vi "saveLogEntry.vi"(8 "error in (no error)":errorcluster, 11 "Logger in":refnum<class "TestDataLog.lvclass">) -> (0 "error out":errorcluster, 3 "Logger out":refnum<class "TestDataLog.lvclass">)   [LabVIEW 2015, in "TestDataLog.lvclass"]
uses:
  TestDataLog.lvclass
  TestDataLog.lvclass/TestDataLog.ctl
  <userlib>/Common/Log/Log/Log.lvclass/Log.ctl
  <userlib>/Common/Log/Log/Log.lvclass
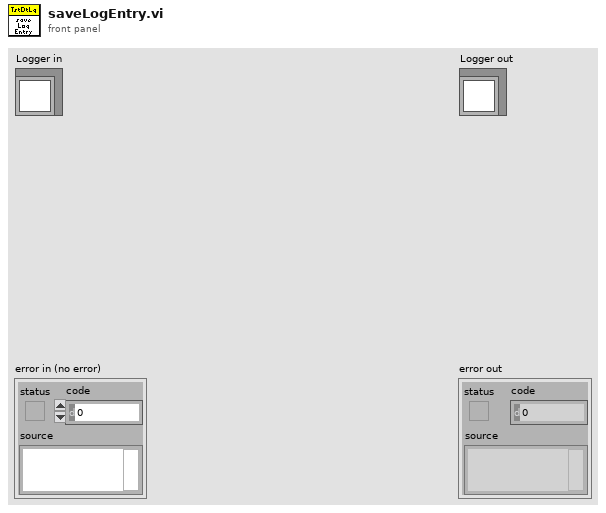
[diagram p1: front panel]
types:
  T1 = typedef "M1M3SSSTypedefs.lvlib/InputData.ctl" = cluster{"Force Measured":T2, "Distance Data":T3}
  T2 = typedef "M1M3SSSTypedefs.lvlib/ForceDemand.ctl" = dbl[unit]
  T3 = typedef "DistanceGauge.lvlib/Distance Data.ctl" = cluster{"Distance Measured 1":dbl[unit], "Distance Measured 2":dbl[unit]}
  T4 = typedef "M1M3SSSTypedefs.lvlib/OutputData.ctl" = cluster{"Ramp Output":u16}
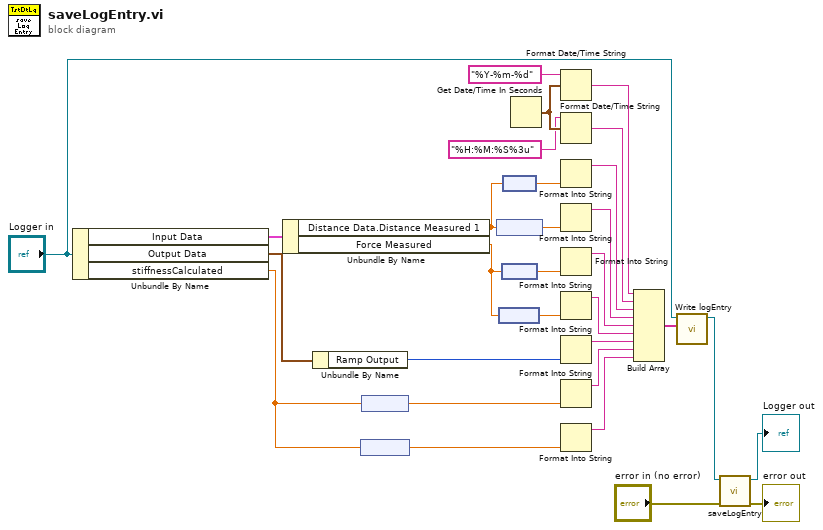
[diagram p0: block diagram]
diagram:
  n1 = Unbundle By Name("Logger in") -> ("Input Data"=w30:T1, "Output Data"=w29:T4, "stiffnessCalculated"=w2:dbl[unit])
  n2 = Unbundle By Name(w30) -> ("Distance Data.Distance Measured 1"=w8:dbl[unit], "Force Measured"=w5:T2)
  n3 = Unbundle By Name(w29) -> ("Ramp Output"=w28:u16)
  n4 = node(w2) -> (w12:dbl)
  n5 = node(w2) -> (w3:dbl)
  n6 = node(w8) -> (w25:dbl)
  n7 = node(w5) -> (w6:dbl)
  n8 = node(w5) -> (w26:dbl)
  n9 = node(w8) -> (w10:dbl)
  n10 = Get Date/Time In Seconds() -> (seconds since 1Jan1904=w24:timestamp)
  n11 = Format Date/Time String(time format string (%c)="%Y-%m-%d" ("format string"), seconds (now)=w24) -> (date/time string=w21:string)  [unwired: 1 in]
  n12 = Format Date/Time String(time format string (%c)="%H:%M:%S%3u", seconds (now)=w24) -> (date/time string=w22:string)  [unwired: 1 in]
  n13 = Format Into String(w10) -> (resulting string=w7:string)  [unwired: 3 in, 1 out]
  n14 = Format Into String(w25) -> (resulting string=w13:string)  [unwired: 3 in, 1 out]
  n15 = Format Into String(w26) -> (resulting string=w14:string)  [unwired: 3 in, 1 out]
  n16 = Format Into String(w6) -> (resulting string=w4:string)  [unwired: 3 in, 1 out]
  n17 = Format Into String(w28) -> (resulting string=w27:string)  [unwired: 3 in, 1 out]
  n18 = Format Into String(w3) -> (resulting string=w1:string)  [unwired: 3 in, 1 out]
  n19 = Format Into String(w12) -> (resulting string=w11:string)  [unwired: 3 in, 1 out]
  n20 = Build Array(w21, w22, w7, w13, w14, w4, w27, w1, w11) -> (w18:string[])
  n21 = call <userlib>:"Write logEntry.vi"("logEntry"=w18, "Logger in"="Logger in") -> ("Logger out"=w19:refnum<class "TestDataLog.lvclass">)  [unwired: 9 in]
  n22 = call-parent "saveLogEntry.vi"("error in (no error)"="error in (no error)", "Logger in"=w19) -> ("error out"=→"error out":errorcluster, "Logger out"=→"Logger out":refnum<class "TestDataLog.lvclass">)  [unwired: 8 in]
